vi "PDE Flexible Element_RHS.vi"(2 "data":variant, 3 "y":dbl, 4 "x":dbl) -> (0 "error out":errorcluster, 1 "F(x, y)":dbl)   [LabVIEW 2023]
doc: "This VI implements the right side of the equation."
panel:
  # "This is an example of a VI that the PDE solver can call by reference. All VIs called by the PDE solver must have the same connector pane."
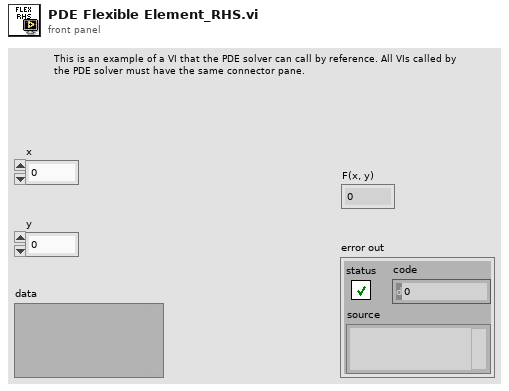
[diagram p1: front panel]
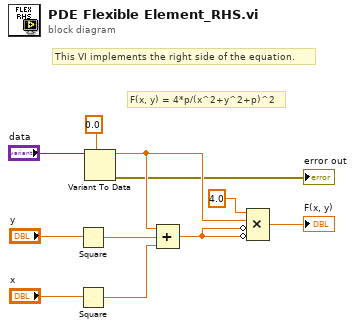
[diagram p0: block diagram]
diagram:
  # "This VI implements the right side of the equation."
  # "F(x, y) = 4*p/(x^2+y^2+p)^2"
  n1 = Square(x="y") -> (x^2=w7:dbl)
  n2 = Square(x="x") -> (x^2=w6:dbl)
  n3 = Variant To Data(type=0.0, Variant="data") -> (data=w3:dbl, error out=→"error out":errorcluster)  [unwired: 1 in]
  n4 = Compound Arithmetic op=ADD(w3, w7, w6) -> (w4:dbl)
  n5 = Compound Arithmetic op=MULTIPLY(4.0 ("value"), w3, invert w4, invert w4) -> (→"F(x, y)":dbl)
